vi "find_stamp_bin.vi"(10 "Histogram_bins":dbl[](array[numeric]), 11 "stamp":i64) -> (2 "out_of_bounds":bool, 3 "bin":i32)   [LabVIEW 2018]
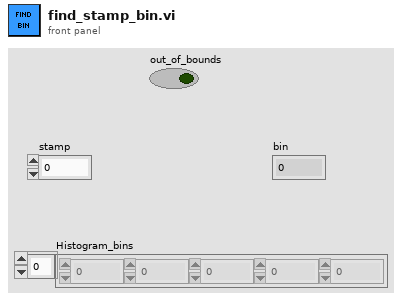
[diagram p1: front panel]
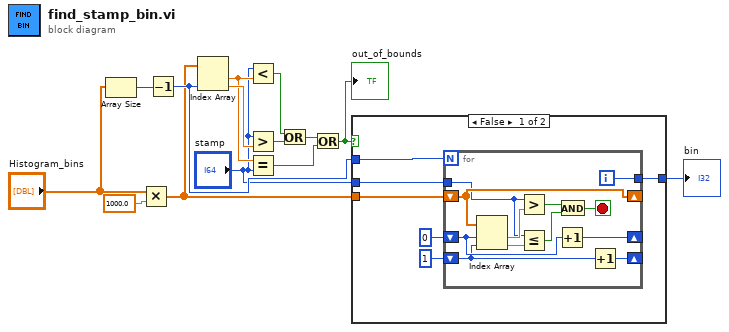
[diagram p0: block diagram]
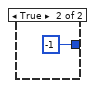
[diagram p2: hidden frame]
diagram:
  n1 = Array Size(array="Histogram_bins") -> (size(s)=w14:i32)
  n2 = Multiply(x="Histogram_bins", y=1000.0) -> (x*y=w1:dbl[])
  n3 = Decrement(x=w14) -> (x-1=w11:i32)
  n4 = Index Array(array=w1, index #2=w11) -> (element #1=w6:dbl, element #2=w10:dbl)  [unwired: 1 in]
  n5 = Less?(x="stamp", y=w6) -> (x < y?=w9:bool)
  n6 = Greater?(x="stamp", y=w10) -> (0:w8:bool)
  n7 = Equal?(x=w6, y="stamp") -> (x = y?=w4:bool)
  n8 = Or(x=w9, y=w8) -> (x .or. y?=w3:bool)
  n9 = Or(x=w3, y=w4) -> (x .or. y?=w2:bool)
  "out_of_bounds" <- w2
  n10 = case shown="False" w2 {
    tunnel: w1 -> [w20 _]
    tunnel: w11 -> [w19 _]
    tunnel: "stamp" -> [w18 _]
    tunnel: [w17 -1] -> w7
    frame False {
      n11 = for {
        N: w19 -> [_]
        tunnel: w18 -> [w30]
        shift-right: [w32] -> _
        shift-left: w20 -> [w32]
        tunnel: [w25] -> w17
        shift-right: [w24] -> _
        shift-left: 0 ("index") -> [w23]
        shift-right: [w21] -> _
        shift-left: 1 ("index") -> [w22]
        i -> [w25]
        stop <- w26 stop-if-true
        n12 = Index Array(array=w32, index #1=w23, index #2=w22) -> (element #1=w31:dbl, element #2=w29:dbl)
        n13 = Greater?(x=w30, y=w31) -> (0:w27:bool)
        n14 = Less Or Equal?(x=w30, y=w29) -> (x <= y?=w28:bool)
        n15 = Increment(x=w23) -> (x+1=w24:i32)
        n16 = And(x=w27, y=w28) -> (x .and. y?=w26:bool)
        n17 = Increment(x=w22) -> (x+1=w21:i32)
      }
    }
    frame True {
    }
  }
  "bin" <- w7
